vi "Read Current step.vi"(8 "error in (no error)":errorcluster, 11 "IV in":refnum<class "IV.lvclass">) -> (0 "error out":errorcluster, 2 "Current step":i32, 3 "IV out":refnum<class "IV.lvclass">)   [LabVIEW 2021, in "IV.lvclass"]
uses:
  IV.lvclass
  IV.lvclass/IV.ctl
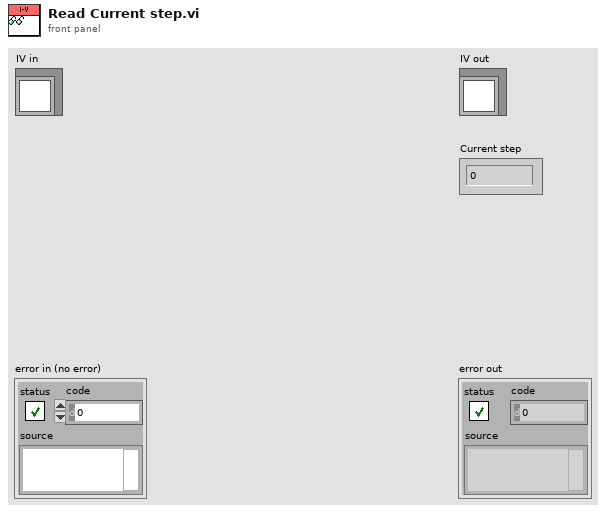
[diagram p1: front panel]
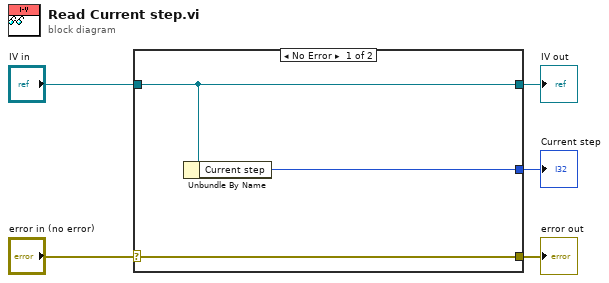
[diagram p0: block diagram]
diagram:
  n1 = case shown="No Error" "error in (no error)" {
    selector: "error in (no error)" -> [w8 w9]
    tunnel: [w8 w9] -> w4
    tunnel: [w7 w10] -> w2
    tunnel: "IV in" -> [w7 w10]
    tunnel: [w6 _] -> w1
    frame No Error {
      n2 = Unbundle By Name(w7) -> ("Current step"=w6:i32)
    }
    frame Error {
    }
  }
  "error out" <- w4
  "IV out" <- w2
  "Current step" <- w1
